vi "SetIdentifier.vi"(8 "error in (no error)":errorcluster, 10 "Identifier":string, 11 "DocumentClass in":refnum<class "Document.lvclass">) -> (0 "error out":errorcluster, 3 "DocumentClass out":refnum<class "Document.lvclass">)   [LabVIEW 2021, in "ProligentXMLGenerator.lvlib" / "Document.lvclass"]
doc: "This document is uniquely identified by its Identifier.\n\nGUID Type."
uses:
  Document.lvclass
  Document.lvclass/Document.ctl
  Base/Guid/Guid.lvclass
  Base/Attribute/Attribute.lvclass
  C:/Projects/proligent-xml-generator-labview/src/ProligentXMLGenerator/Base/NonEmptyString/NonEmptyString.lvclass
  C:/Projects/proligent-xml-generator-labview/src/ProligentXMLGenerator/Base/String/String.lvclass
  C:/Projects/proligent-xml-generator-labview/src/ProligentXMLGenerator/Base/Attribute/Attribute.lvclass
  C:/Projects/proligent-xml-generator-labview/src/ProligentXMLGenerator/Base/Guid/Guid.lvclass
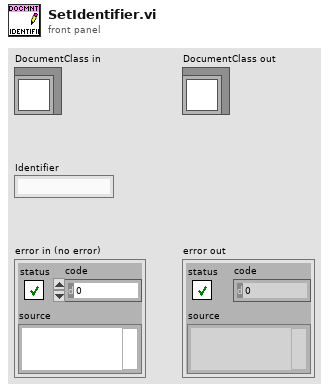
[diagram p1: front panel]
types:
  T1 = typedef "ProligentXMLGenerator.lvlib/Document.lvclass/Data.ctl" = cluster{"Name":string, "CustomData":refnum<class "CustomData.lvclass">, "Identifier":refnum<class "Guid.lvclass">, "NameType":refnum<class "NonEmptyString_255.lvclass">, "FileName":refnum<class "NonEmptyString_255.lvclass">, "Description":refnum<class "NonNullableString_600.lvclass">, "FilePath":path, "DestinationFolder":path}
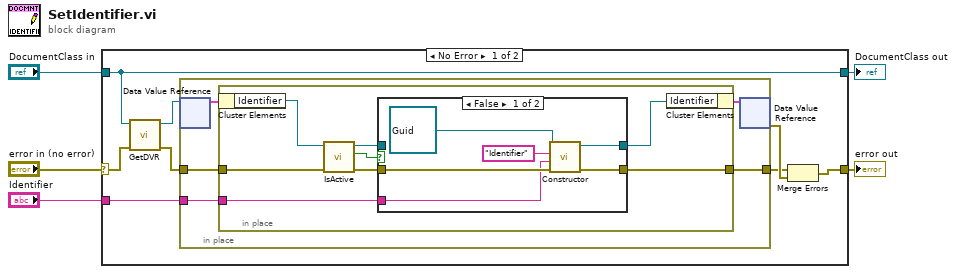
[diagram p0: block diagram]
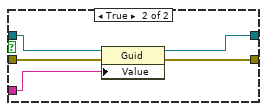
[diagram p2: hidden frame]
diagram:
  n1 = case shown="No Error" "error in (no error)" {
    selector: "error in (no error)" -> [w11 w38]
    tunnel: "DocumentClass in" -> [w7 w39]
    tunnel: [w9 w38] -> w2
    tunnel: "Identifier" -> [w8 _]
    tunnel: [w7 w39] -> w4
    frame No Error {
      n2 = call "GetDVR.vi"("error in"=w11, "Document in"=w7) -> ("error out"=w10:errorcluster, "DVRReference"=w12:refnum<data-value>)  [unwired: 8 in]
      n3 = in-place "In Place Element Structure" {
        in-place-border: w10 -> [w18]
        in-place-border: w8 -> [w17]
        in-place-border: [w14] -> w6
        n4 = in-place-dvr #1(w12) -> (w16:T1)  [unwired: 1 out]
        n5 = in-place "In Place Element Structure" {
          in-place-border: w18 -> [w22]
          in-place-border: w17 -> [w19]
          in-place-border: [w20] -> w14
          n6 = in-place-cluster #2(w16) -> ("Identifier"=w23:refnum<class "Guid.lvclass">)
          n7 = call "IsActive.vi"("error in"=w22, "Attribute in"=w23) -> ("error out"=w26:errorcluster, "IsActive"=w24:bool, "Attribute in"=w25:refnum<class "Guid.lvclass">)  [unwired: 7 in]
          n8 = case shown="False" w24 {
            tunnel: w26 -> [w29 w37]
            tunnel: [w32 w36] -> w20
            tunnel: w19 -> [w28 w35]
            tunnel: [w31 w34] -> w21
            tunnel: w25 -> [_ w33]
            frame False {
              n9 = call-dynamic "Constructor.vi"("error in"=w29, "Value"=w28, "Name"="Identifier", "String in"=refnum<class "Guid.lvclass"> refnum ("ProcessVersion")) -> ("error out"=w32:errorcluster, "String out"=w31:refnum<class "Guid.lvclass">)  [unwired: 6 in]
            }
            frame True {
              n10 = property on="Property Node" class="Guid"(reference=w33, error in=w37, "Value"=w35) -> (reference out=w34:refnum<class "Guid.lvclass">, error out=w36:errorcluster)
            }
          }
          n11 = in-place-cluster #2("Identifier"=w21) -> (w15:T1)
        }
        n12 = in-place-dvr #1(w15) -> (w13:errorcluster)  [unwired: 1 out]
      }
      n13 = Merge Errors(w6, w13) -> (w9:errorcluster)
    }
    frame Error {
    }
  }
  "error out" <- w2
  "DocumentClass out" <- w4
